vi "Apply calib tool box values to main gui.vi"(8 "error in (no error)":errorcluster, 11 "Calibration GUI parameters in":T2) -> (0 "error out":errorcluster, 2 "Current Objective":string, 3 "Updated frame size":T1=200 items=["100X100"=100, "128X128"=128, "200X200"=200, "256X256"=256, "512X512"=512, "1024x1024"=1024, "2048x2048"=2048])   [LabVIEW 2020]
uses:
  TypeDefs/Calibration GUI parameter refs.ctl
  Typedefs/Frame Size.ctl
  Global Variables/gl_UI Ctrl Refs.vi
  Typedefs/Objective selector control enum.ctl
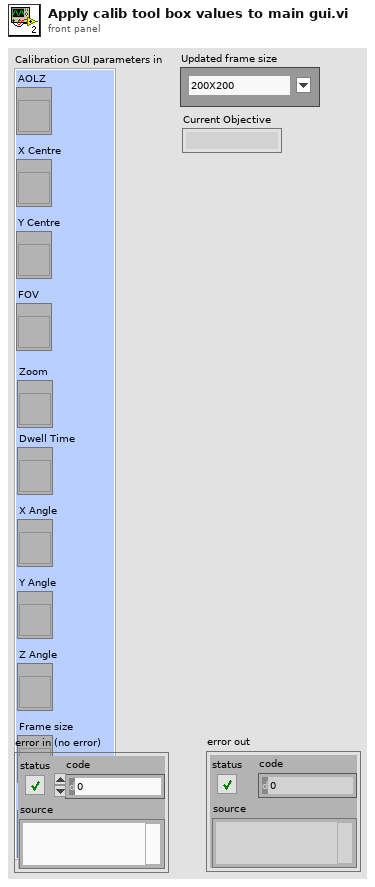
[diagram p1: front panel]
types:
  T1 = typedef "Frame Size.ctl" = u16
  T2 = typedef "Calibration GUI parameter refs.ctl" = cluster{"AOLZ":refnum<vi>, "X Centre":refnum<vi>, "Y Centre":refnum<vi>, "FOV":refnum<vi>, "Dwell Time":refnum<vi>, "X Angle":refnum<vi>, "Y Angle":refnum<vi>, "Z Angle":refnum<vi>, "Frame size":refnum<vi>, "Current Objective":refnum<vi>, "Zoom":refnum<vi>}
  T3 = typedef "UI ctrl refs cluster.ctl" = cluster{"Top level VI path":path, "Top level VI ref":refnum<vi>, "User menu ref":refnum<k9>, "Sub Panel control":refnum<vi>, "Imaging Param Tab":refnum<vi>, "Occurrence-Start drivers":refnum<k4>, "Occurrence-Speed logging initialised":refnum<k4>, "Occurrence-XYZ stage initialised":refnum<k4>, "Exit button":refnum<vi>, "Status ind":refnum<vi>, "Set as origin":refnum<vi>, "Speed Logging":refnum<vi>, "Time Lapse":refnum<vi>, "Live Imaging":refnum<vi>, "AOL Z Stack":refnum<vi>, "Motor Z Stack":refnum<vi>, "Funct Acq button":refnum<vi>, "Hard Shutter":refnum<vi>, "Virtual Shutter":refnum<vi>, "Laser Power":refnum<vi>, "AOL Mode":refnum<vi>, "Frame Size":refnum<vi>, "Field of View":refnum<vi>, "Dwell Time":refnum<vi>, "Zoom":refnum<vi>, "AOL Z":refnum<vi>, "Objective":refnum<vi>, "Axis":refnum<vi>, "Paths & Names":refnum<vi>, "Experiment folder path (ind.)":refnum<vi>, "Last State (Ind.)":refnum<vi>, "Averages":refnum<vi>, "Angle (degrees)":refnum<vi>, "X centre":refnum<vi>, "Y centre":refnum<vi>, "Plane Mode":refnum<vi>, "# Planes":refnum<vi>, "Z Start":refnum<vi>, "Z Stop":refnum<vi>, "Z Step":refnum<vi>, "PMT 1":refnum<vi>, "PMT 2":refnum<vi>, "Stage XYZ Position":refnum<vi>, "Pockels@Z Start":refnum<vi>, "Pockels@Z Stop":refnum<vi>, "Obtain Z Start":refnum<vi>, "Obtain Z Stop":refnum<vi>, "Live stim.trig.period":refnum<vi>, "Live stim.trig.enable":refnum<vi>, "Movement Correction":refnum<vi>, "Load Reference Image":refnum<vi>, "XY Stage Move":refnum<vi>, "MovCor Cluster":refnum<vi>, "RefDAQParam":refnum<vi>, "Funct. Acq. Pockels Modulation":refnum<vi>, "Ref Laser Power":refnum<vi>, "Enable Video Recording":refnum<vi>, "Video Record-Live Imaging":refnum<vi>, "Video Record-Funct acq":refnum<vi>, "Reference Source":refnum<vi>, "AOL Z-stack Chirps Ready (ind)":refnum<vi>, "Target time between mov.cor. ref triggers (ms)":refnum<vi>, "Funct. Acq. Ref frame save":refnum<vi>, "Tracking button":refnum<vi>, "Show ref plots window":refnum<vi>, "Center freq ind (nm)":refnum<vi>, "Pickup mode (ind)":refnum<vi>, "Logging queue (ind)":refnum<vi>, "Back aperture power (ind.)":refnum<vi>, "Power after objective (ind.)":refnum<vi>, "Switch user":refnum<vi>, "Ls1 Conn. Status":refnum<vi>, "Ls1Tuning Status":refnum<vi>, "Ls1 Faults":refnum<vi>, "Ls1 Connection":refnum<vi>, "Ls1 Mode":refnum<vi>, "Ls1 POWER [mW]":refnum<vi>, "Ls1Shutter":refnum<vi>, "Ls1 Wavelength":refnum<vi>, "Ls1 Note":refnum<vi>, "Ls1 Confirm Wav":refnum<vi>, "Ls1 PreChrp Prism1":refnum<vi>, "Ls1 PreChrp Prism2":refnum<vi>, "Ls1 wav top Ind":refnum<vi>, "Ls1 power top Ind":refnum<vi>, "Ls1 Pump peak Hold":refnum<vi>, "Ls1 Status Ind":refnum<vi>, "Ls1 wav cancel":refnum<vi>, "Experiment Type":refnum<vi>, "Biology Information":refnum<vi>}
  T4 = typedef "Plane Mode.ctl" = u16
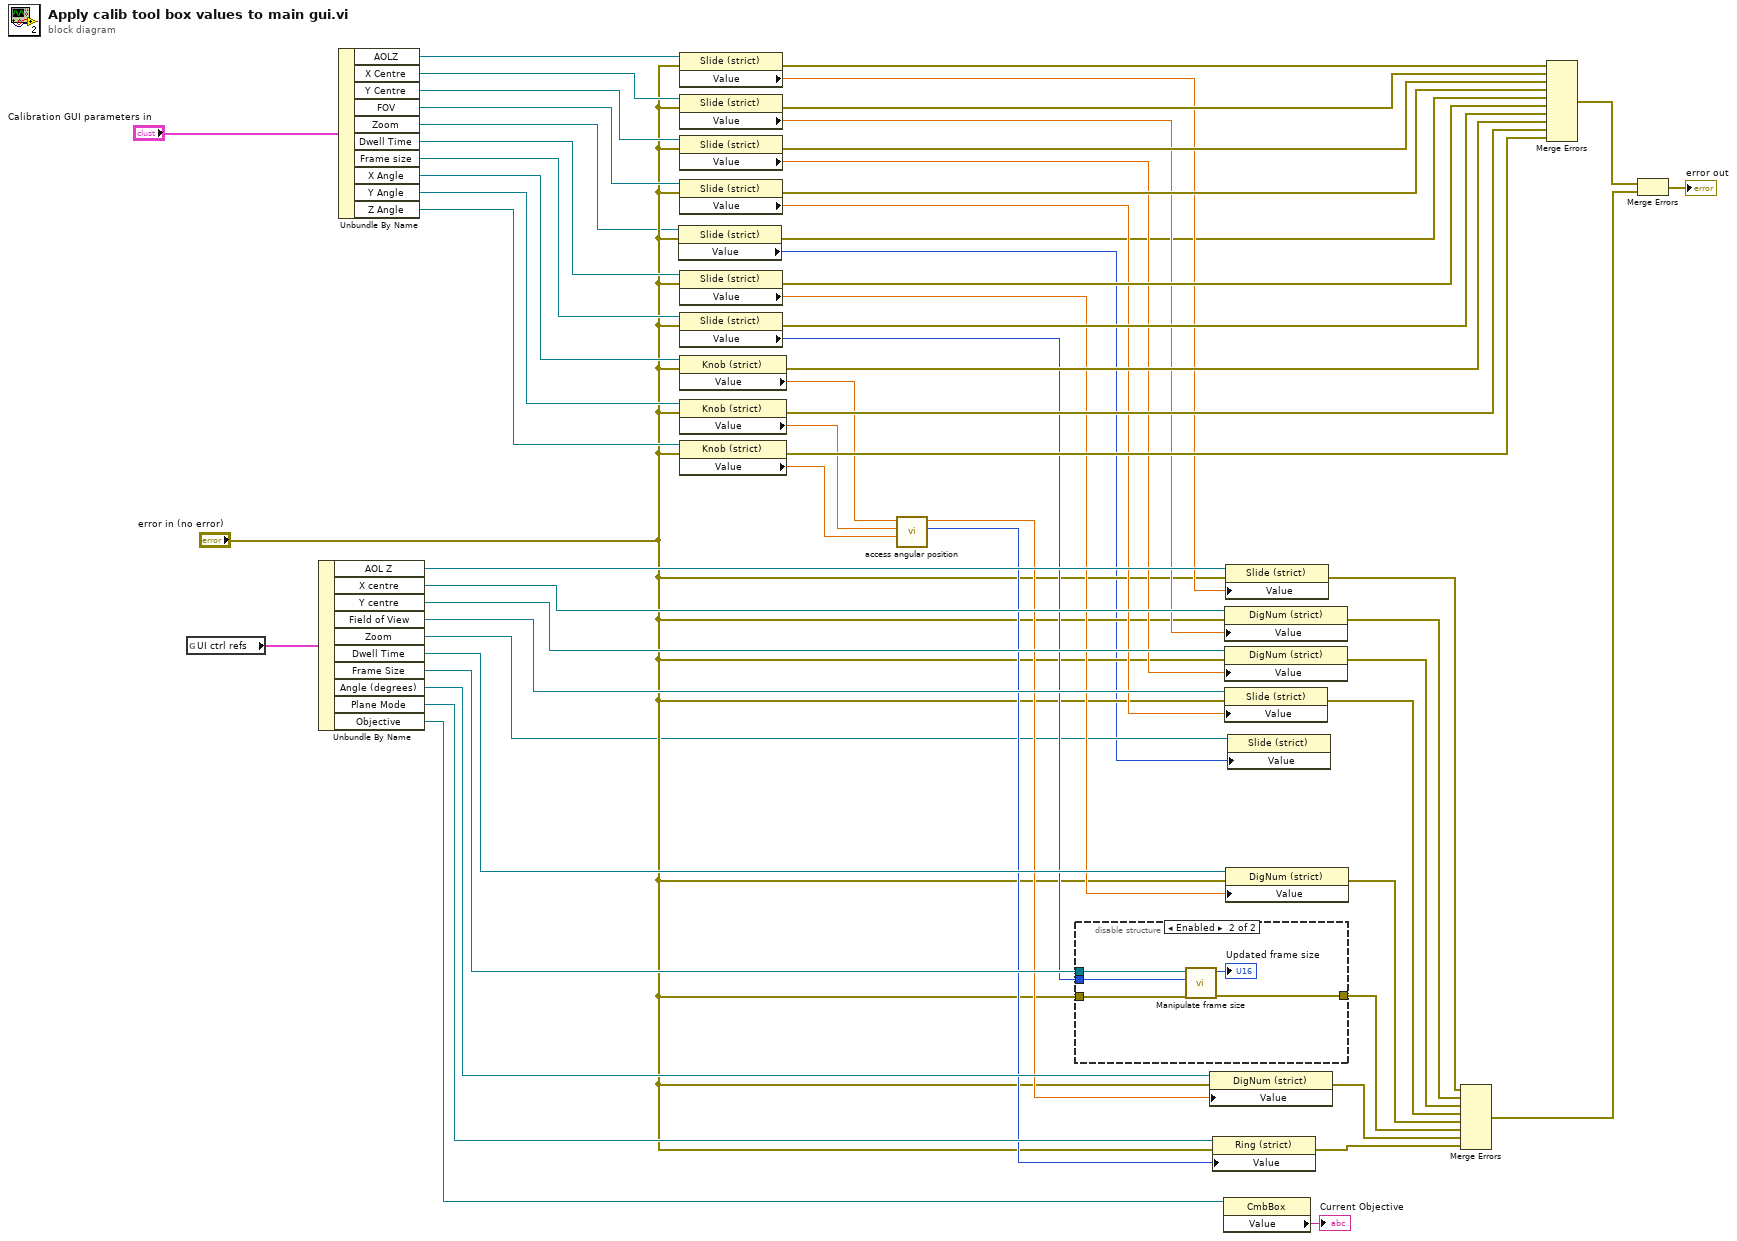
[diagram p0: block diagram]
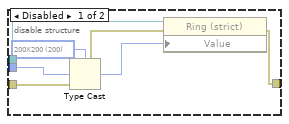
[diagram p2: hidden frame]
diagram:
  n1 = global read "gl_UI Ctrl Refs.vi" "UI ctrl refs"() -> (w57:T3)
  n2 = Unbundle By Name(w57) -> ("AOL Z"=w49:refnum<vi>, "X centre"=w48:refnum<vi>, "Y centre"=w47:refnum<vi>, "Field of View"=w46:refnum<vi>, "Zoom"=w2:refnum<vi>, "Dwell Time"=w45:refnum<vi>, "Frame Size"=w42:refnum<vi>, "Angle (degrees)"=w44:refnum<vi>, "Plane Mode"=w43:refnum<vi>, "Objective"=w7:refnum<vi>)
  n3 = Unbundle By Name("Calibration GUI parameters in") -> ("AOLZ"=w55:refnum<vi>, "X Centre"=w54:refnum<vi>, "Y Centre"=w53:refnum<vi>, "FOV"=w52:refnum<vi>, "Zoom"=w3:refnum<vi>, "Dwell Time"=w51:refnum<vi>, "Frame size"=w50:refnum<vi>, "X Angle"=w41:refnum<vi>, "Y Angle"=w40:refnum<vi>, "Z Angle"=w39:refnum<vi>)
  n4 = property class="Slide (strict)"(reference=w3, error in="error in (no error)") -> (error out=w4:errorcluster, "Value"=w1:i8)  [unwired: 1 out]
  n5 = property class="Slide (strict)"(reference=w55, error in="error in (no error)") -> (error out=w30:errorcluster, "Value"=w18:sgl)  [unwired: 1 out]
  n6 = property class="Slide (strict)"(reference=w54, error in="error in (no error)") -> (error out=w29:errorcluster, "Value"=w17:sgl)  [unwired: 1 out]
  n7 = property class="Slide (strict)"(reference=w53, error in="error in (no error)") -> (error out=w28:errorcluster, "Value"=w16:sgl)  [unwired: 1 out]
  n8 = property class="Slide (strict)"(reference=w52, error in="error in (no error)") -> (error out=w27:errorcluster, "Value"=w15:sgl)  [unwired: 1 out]
  n9 = property class="Slide (strict)"(reference=w51, error in="error in (no error)") -> (error out=w26:errorcluster, "Value"=w14:dbl)  [unwired: 1 out]
  n10 = property class="Slide (strict)"(reference=w50, error in="error in (no error)") -> (error out=w25:errorcluster, "Value"=w13:u16)  [unwired: 1 out]
  n11 = property class="Knob (strict)"(reference=w41, error in="error in (no error)") -> (error out=w24:errorcluster, "Value"=w12:dbl)  [unwired: 1 out]
  n12 = property class="Knob (strict)"(reference=w40, error in="error in (no error)") -> (error out=w23:errorcluster, "Value"=w11:dbl)  [unwired: 1 out]
  n13 = property class="Knob (strict)"(reference=w39, error in="error in (no error)") -> (error out=w22:errorcluster, "Value"=w10:dbl)  [unwired: 1 out]
  n14 = call "access angular position.vi"("Z angle"=w10, "Y angle"=w11, "x angle"=w12) -> ("Value"=w8:T4, "Angle"=w9:dbl)  [unwired: 7 in]
  n15 = disable-structure shown="Enabled" {
    disable-tunnel: w42 -> [w63 w68]
    disable-tunnel: [w62 w65] -> w33
    disable-tunnel: "error in (no error)" -> [w61 w66]
    disable-tunnel: w13 -> [w59 w67]
    frame Disabled {
      w60 = T1 200 items=["100X100"=100, "128X128"=128, "200X200"=200, "256X256"=256, "512X512"=512, "1024x1024"=1024, "2048x2048"=2048] ("Value")
      n16 = Type Cast(type=w60, x=w59) -> (*(type *) &x=w58:T1)
      n17 = property class="Ring (strict)"(reference=w63, error in=w61, "Value"=w58) -> (error out=w62:errorcluster)  [unwired: 1 out]
    }
    frame Enabled {
      n18 = call "Manipulate frame size.vi"("error in (no error)"=w66, "Value"=w67, "Frame Size"=w68) -> ("error out"=w65:errorcluster, "Updated frame size"=→"Updated frame size":T1)  [unwired: 7 in]
    }
  }
  n19 = property class="DigNum (strict)"(reference=w44, error in="error in (no error)", "Value"=w9) -> (error out=w32:errorcluster)  [unwired: 1 out]
  n20 = property class="Ring (strict)"(reference=w43, error in="error in (no error)", "Value"=w8) -> (error out=w31:errorcluster)  [unwired: 1 out]
  n21 = property class="CmbBox"(reference=w7) -> ("Value"=→"Current Objective":string)  [unwired: 1 in, 2 out]
  n22 = property class="DigNum (strict)"(reference=w48, error in="error in (no error)", "Value"=w17) -> (error out=w37:errorcluster)  [unwired: 1 out]
  n23 = property class="DigNum (strict)"(reference=w47, error in="error in (no error)", "Value"=w16) -> (error out=w36:errorcluster)  [unwired: 1 out]
  n24 = property class="Slide (strict)"(reference=w46, error in="error in (no error)", "Value"=w15) -> (error out=w35:errorcluster)  [unwired: 1 out]
  n25 = property class="Slide (strict)"(reference=w49, error in="error in (no error)", "Value"=w18) -> (error out=w38:errorcluster)  [unwired: 1 out]
  n26 = property class="DigNum (strict)"(reference=w45, error in="error in (no error)", "Value"=w14) -> (error out=w34:errorcluster)  [unwired: 1 out]
  n27 = property class="Slide (strict)"(reference=w2, "Value"=w1) -> ()  [unwired: 1 in, 2 out]
  n28 = Merge Errors(w38, w37, w36, w35, w34, w33, w32, w31) -> (w20:errorcluster)
  n29 = Merge Errors(w30, w29, w28, w27, w4, w26, w25, w24, w23, w22) -> (w21:errorcluster)
  n30 = Merge Errors(w21, w20) -> (→"error out":errorcluster)
